vi "Periodic Tasks.vi"() -> ()   [LabVIEW 2011]
doc: "This VI runs in parallel to other tasks. It can contain as many user-defined periodic loops as you need. These can carry out PID or other sorts of timed response."
uses:
  <vilib>/Platform/TimedLoop/XDataNode/timing_clust.ctl
  <vilib>/Platform/TimedLoop/XDataNode/nitl_modes.ctl
  <vilib>/Platform/TimedLoop/XDataNode/wakeup.ctl
  <vilib>/Rock Robotics/WPI/Ultrasonic/WPI_UltrasonicRangeUnits.ctl
  Robot Global Data.vi
  <vilib>/Platform/TimedLoop/XDataNode/XDataNode.xnode
  <vilib>/Platform/TimedLoop/XDataNode/XDNodeRunTimeDep.lvlib
panel:
  out "Angle 2":dbl
  out "Forward Distance":dbl
  in  "pingtime (Sec) 2":sgl=0.5
  out "Angle":dbl
  in  "pingtime (Sec)":sgl=0.5
  out "Ultrasonic Distance":dbl
  # "Outputs"
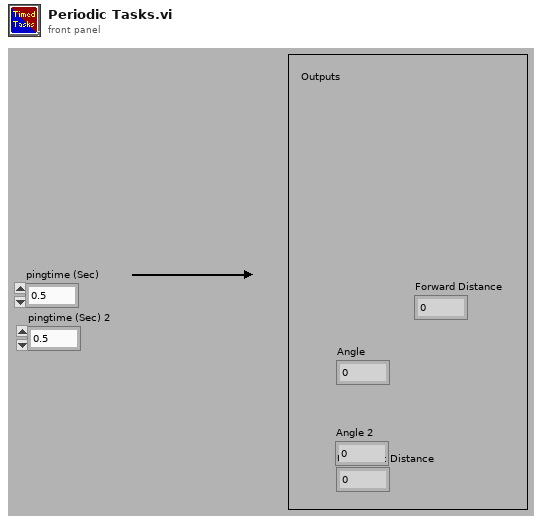
[diagram p1: front panel]
types:
  T1 = typedef "WPI_GyroDevRef.ctl" = cluster{"DevStatus":errorcluster, "Analog Module":T2, "Analog Channel":T3, "Offset":dbl, "Gain (VoltsPerDegree/Second)":dbl}
  T2 = typedef "FPGA_TypedefAnalogModule.ctl" = enum16{"Analog Module 1", "Analog Module 2"}
  T3 = typedef "FPGA_AIChannel.ctl" = enum8{"AI 1", "AI 2", "AI 3", "AI 4", "AI 5", "AI 6", "AI 7", "AI 8", "Invalid"}
  T4 = typedef "WPI_SerialPortRef.ctl" = cluster{"DevStatus":errorcluster, "Serial Port Name":refnum<visa-resource-name>}
  T5 = typedef "WPI_EncoderDevRef.ctl" = cluster{"DevStatus":errorcluster, "EncoderIndex":T6, "CounterIndex":T7, "DistancePerCount":dbl, "Decoding Type":T8}
  T6 = typedef "FPGA_EncoderIdx.ctl" = enum8{"Enc 0", "Enc 1", "Enc 2", "Enc 3", "Invalid"}
  T7 = typedef "FPGA_CounterCtrSystemIndex.ctl" = enum8{"Ctr 0", "Ctr 1", "Ctr 2", "Ctr 3", "Ctr 4", "Ctr 5", "Ctr 6", "Ctr 7", "Invalid"}
  T8 = typedef "WPI_EncoderType.ctl" = enum16{"1x", "2x", "4x"}
  T9 = typedef "WPI_UltrasonicDeviceRef.ctl" = cluster{"DevStatus":errorcluster, "Ping Digital Module":T10, "Echo Digital Module":T10, "Ping Channel":T11, "Echo Channel":T11, "CntIndex":T7}
  T10 = typedef "FPGA_TypedefDigitalModule.ctl" = enum16{"Digital Module 1", "Digital Module 2"}
  T11 = typedef "FPGA_DIOChannel.ctl" = enum8{"DIO 1", "DIO 2", "DIO 3", "DIO 4", "DIO 5", "DIO 6", "DIO 7", "DIO 8", "DIO 9", "DIO 10", "DIO 11", "DIO 12", "DIO 13", "DIO 14", "Invalid"}
  T12 = typedef "WPI_RelayDevRef.ctl" = cluster{"DevStatus":errorcluster, "Relay Channel":T13, "Digital Module":T10, "Relay Direction":T14}
  T13 = typedef "FPGA_DIORelayChannel.ctl" = enum8{"Relay 1", "Relay 2", "Relay 3", "Relay 4", "Relay 5", "Relay 6", "Relay 7", "Relay 8", "Invalid"}
  T14 = typedef "WPI_RelayDirection.ctl" = enum16{"Both directions", "Forward only", "Reverse only"}
  T15 = typedef "XDNodeRunTimeDep.lvlib/timing_clust.ctl" = cluster{"Expected End [f-1]":u64, "Actual End [f-1]":u64, "Finished Late? [f-1]":bool, "Expected End [i-1]":u64, "Actual End [i-1]":u64, "Finished Late? [i-1]":bool, "Expected Start [i]":u64, "Actual Start [i]":u64, "Expected Start [f]":u64, "Actual Start [f]":u64, "Source Name":string, "Structure Name":string, "Period":i64, "Deadline":i64, "Offset":i64, "Start":i64, "Priority":i32, "Timeout":i32, "Mode":T16, "Wakeup Reason":T17, "Error":errorcluster, "Source Type":string, "Secondary Source Type":string, "Global End Time":u64, "Global Start Time":u64, "Frame Duration":u64, "Iteration Duration":u64, "Assigned CPU":i32, "I/O Scan Engine Mode":u32}
  T16 = typedef "XDNodeRunTimeDep.lvlib/nitl_modes.ctl" = enum32{"No Change", "Process missed periods, maintain original phase", "Discard missed periods, maintain original phase", "Process missed periods, ignore original phase", "Discard missed periods, ignore original phase"}
  T17 = typedef "XDNodeRunTimeDep.lvlib/wakeup.ctl" = enum32{"Normal", "Aborted", "Asynchronous wakeup", "Timing source error", "Timed loop error", "Timeout"}
  T18 = typedef "WPI_UltrasonicRangeUnits.ctl" = enum16{"inches", "mm"}
  T19 = cluster{"Driver Station Digital Input (1-8)[0]":bool, "Driver Station Digital Input (1-8)[1]":bool, "Driver Station Digital Input (1-8)[2]":bool, "Driver Station Digital Input (1-8)[3]":bool, "Driver Station Digital Input (1-8)[4]":bool, "Driver Station Digital Input (1-8)[5]":bool, "Driver Station Digital Input (1-8)[6]":bool, "Driver Station Digital Input (1-8)[7]":bool, "Driver Station Digital Input (1-8)[8]":bool}
  T20 = cluster{"Axis 1":dbl, "Axis 2":dbl, "Axis 3":dbl, "Axis 4":dbl, "Axis 5":dbl, "Axis 6":dbl, "Button 1":bool, "Button 2":bool, "Button 3":bool, "Button 4":bool, "Button 5":bool, "Button 6":bool, "Button 7":bool, "Button 8":bool, "Button 9":bool, "Button 10":bool, "Button 11":bool, "Button 12":bool}
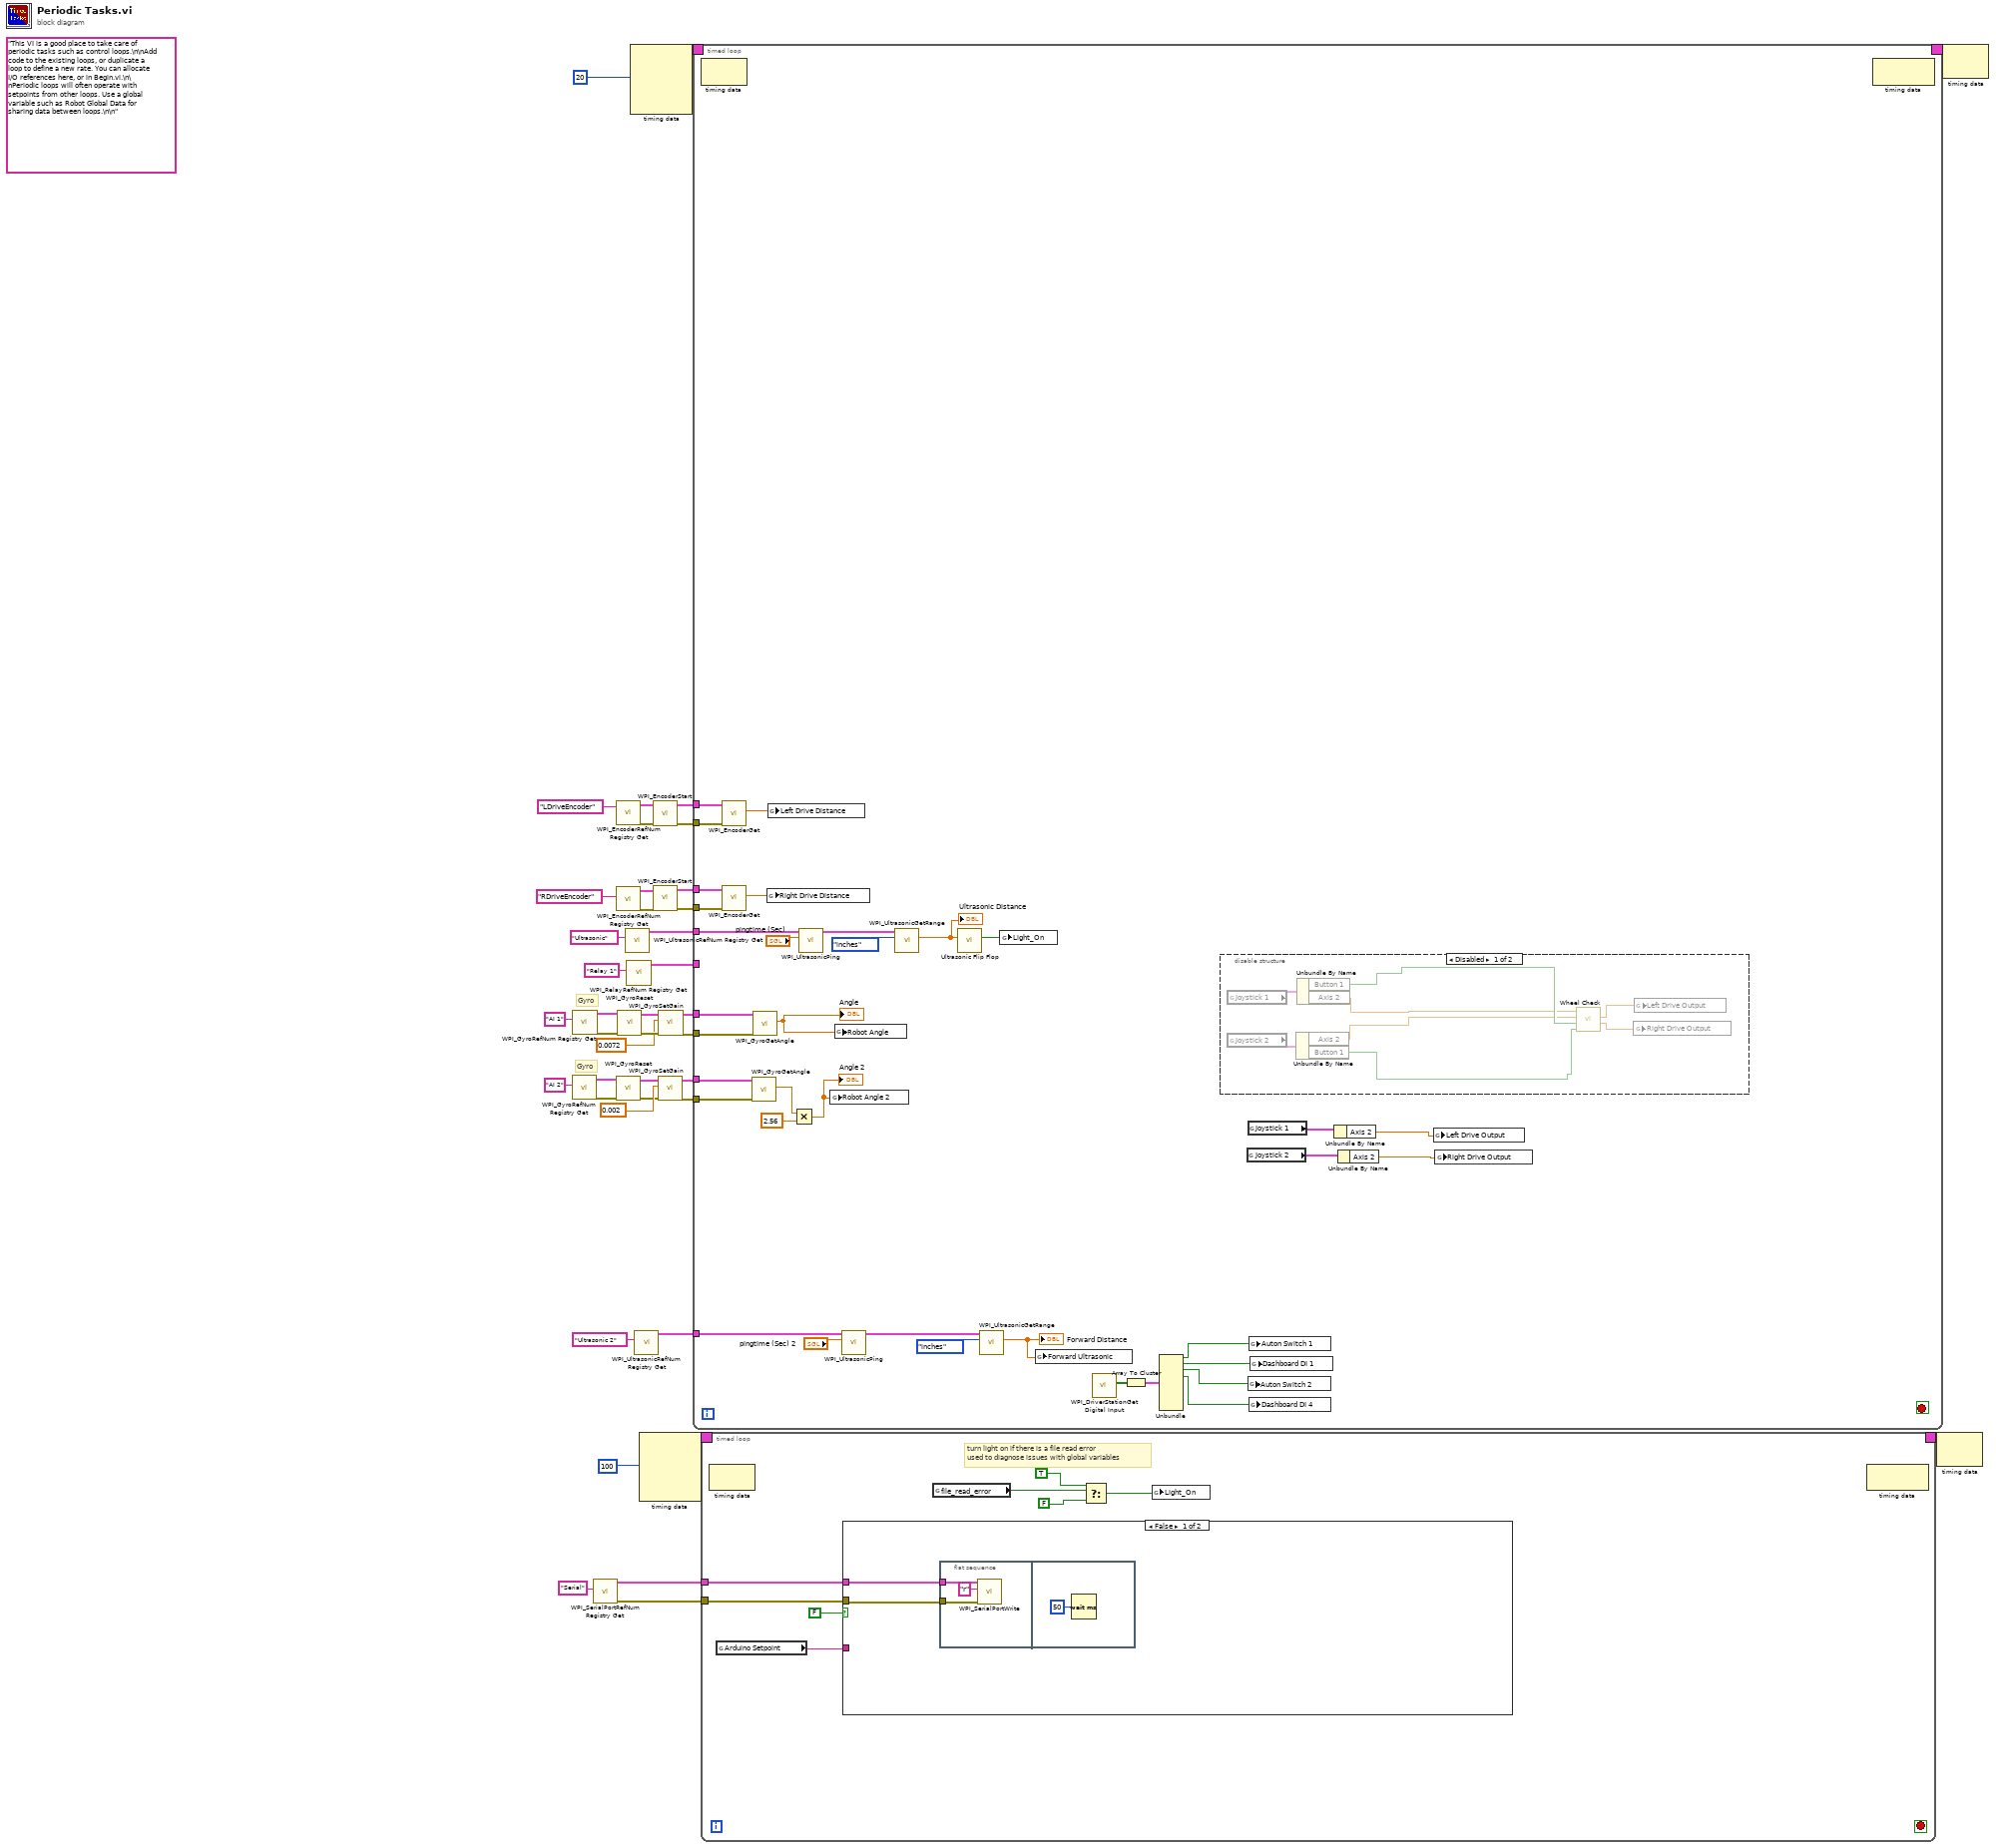
[diagram p0: block diagram]
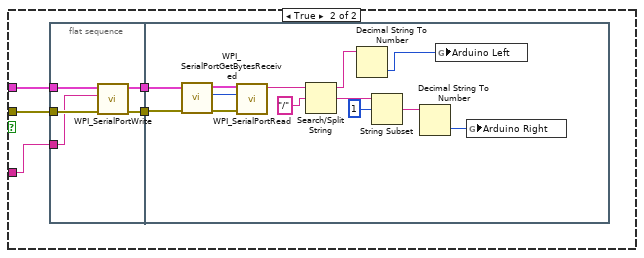
[diagram p2: hidden frame]
diagram:
  (unwired) "This VI is a good place to take care of periodic tasks such as control loops.\n\nAdd code to the existing loops, or duplicate a loop to define a new rate. You can allocate I/O references here, or in Begin.vi.\n\nPeriodic loops will often operate with setpoints from other loops. Use a global variable such as Robot Global Data for sharing data between loops.\n\n"
  # "Gyro"
  # "Gyro"
  n1 = call <vilib>:"WPI_GyroRefNum Registry Get.vi"("refnum name"="AI 2") -> ("error out"=w1:errorcluster, "GyroDevRef"=w8:T1)  [unwired: 1 in, 8 out]
  n2 = call <vilib>:"WPI_GyroRefNum Registry Get.vi"("refnum name"="AI 1") -> ("error out"=w24:errorcluster, "GyroDevRef"=w17:T1)  [unwired: 1 in, 8 out]
  n3 = call <vilib>:"WPI_SerialPortRefNum Registry Get.vi"("refnum name"="Serial") -> ("error out"=w25:errorcluster, "SerialPortRef"=w26:T4)  [unwired: 1 in, 8 out]
  n4 = call <vilib>:"WPI_EncoderRefNum Registry Get.vi"("refnum name"="LDriveEncoder") -> ("error out"=w10:errorcluster, "EncoderDevRef"=w11:T5)  [unwired: 1 in, 8 out]
  n5 = call <vilib>:"WPI_EncoderRefNum Registry Get.vi"("refnum name"="RDriveEncoder") -> ("error out"=w12:errorcluster, "EncoderDevRef"=w13:T5)  [unwired: 1 in, 8 out]
  n6 = call <vilib>:"WPI_GyroReset.vi"("error in (no error)"=w1, "GyroDevRef"=w8) -> ("error out"=w3:errorcluster, "GyroDevRef"=w4:T1)  [unwired: 8 out]
  n7 = call <vilib>:"WPI_GyroReset.vi"("error in (no error)"=w24, "GyroDevRef"=w17) -> ("error out"=w22:errorcluster, "GyroDevRef"=w21:T1)  [unwired: 8 out]
  n8 = call <vilib>:"WPI_UltrasonicRefNum Registry Get.vi"("refnum name"="Ultrasonic") -> ("UltrasonicDevRef"=w28:T9)  [unwired: 1 in, 9 out]
  n9 = call <vilib>:"WPI_RelayRefNum Registry Get.vi"("refnum name"="Relay 1") -> ("RelayDevRef"=w41:T12)  [unwired: 1 in, 9 out]
  n10 = node-c288(i64 20 ("Period")) -> (w39:T15)  [unwired: 3 out]
  n11 = call <vilib>:"WPI_UltrasonicRefNum Registry Get.vi"("refnum name"="Ultrasonic 2") -> ("UltrasonicDevRef"=w16:T9)  [unwired: 1 in, 9 out]
  n12 = node-c288(i64 100 ("Period")) -> (w36:T15)  [unwired: 3 out]
  n13 = call <vilib>:"WPI_EncoderStart.vi"("error in (no error)"=w10, "EncoderDevRef"=w11) -> ("error out"=w33:errorcluster, "EncoderDevRef"=w32:T5)  [unwired: 8 out]
  n14 = call <vilib>:"WPI_EncoderStart.vi"("error in (no error)"=w12, "EncoderDevRef"=w13) -> ("error out"=w30:errorcluster, "EncoderDevRef"=w31:T5)  [unwired: 8 out]
  n15 = call <vilib>:"WPI_GyroSetGain.vi"("error in (no error)"=w3, "Gain (VoltsPerDegree/Second)"=0.002, "GyroDevRef"=w4) -> ("error out"=w6:errorcluster, "GyroDevRef"=w5:T1)  [unwired: 7 out]
  n16 = call <vilib>:"WPI_GyroSetGain.vi"("error in (no error)"=w22, "Gain (VoltsPerDegree/Second)"=0.0072, "GyroDevRef"=w21) -> ("error out"=w19:errorcluster, "GyroDevRef"=w20:T1)  [unwired: 7 out]
  n17 = timed-loop {
    tunnel: w41 -> [_]
    timing: w39 -> [_]
    timing-out: [_] -> w38
    tunnel: w33 -> [w69]
    tunnel: w32 -> [w70]
    tunnel: w30 -> [w67]
    tunnel: w31 -> [w68]
    tunnel: w28 -> [w73]
    tunnel: w20 -> [w66]
    tunnel: w19 -> [w65]
    tunnel: w16 -> [w60]
    tunnel: w5 -> [w49]
    tunnel: w6 -> [w50]
    stop <- _ stop-if-true
    n18 = node-c288() -> ()  [unwired: 2 out]
    n19 = call <vilib>:"WPI_EncoderGet.vi"("error in (no error)"=w69, "EncoderDevRef"=w70) -> ("Distance"=w76:dbl)  [unwired: 9 out]
    n20 = call <vilib>:"WPI_EncoderGet.vi"("error in (no error)"=w67, "EncoderDevRef"=w68) -> ("Distance"=w75:dbl)  [unwired: 9 out]
    n21 = call <vilib>:"WPI_GyroGetAngle.vi"("error in (no error)"=w50, "GyroDevRef"=w49) -> ("Angle"=w47:dbl)  [unwired: 9 out]
    n22 = call <vilib>:"WPI_GyroGetAngle.vi"("error in (no error)"=w65, "GyroDevRef"=w66) -> ("Angle"=w64:dbl)  [unwired: 9 out]
    "Angle" <- w64
    n23 = global write "Robot Global Data.vi" "Right Drive Distance"(w75) -> ()
    n24 = global write "Robot Global Data.vi" "Left Drive Distance"(w76) -> ()
    n25 = Multiply(x=w47, y=2.56) -> (x*y=w46:dbl)
    "Angle 2" <- w46
    n26 = call <vilib>:"WPI_UltrasonicPing.vi"("pingtime (Sec)"="pingtime (Sec)", "UltrasonicDevRef"=w73) -> ("UltrasonicDevRef"=w72:T9)  [unwired: 1 in, 8 out]
    n27 = global write "Robot Global Data.vi" "Robot Angle 2"(w46) -> ()
    n28 = global write "Robot Global Data.vi" "Robot Angle"(w64) -> ()
    n29 = call <vilib>:"WPI_UltrasonicPing.vi"("pingtime (Sec)"="pingtime (Sec) 2", "UltrasonicDevRef"=w60) -> ("UltrasonicDevRef"=w61:T9)  [unwired: 1 in, 8 out]
    n30 = call <vilib>:"WPI_UltrasonicGetRange.vi"("Range Units"=WPI_UltrasonicRangeUnits."inches", "UltrasonicDevRef"=w72) -> ("Distance"=w63:dbl)  [unwired: 1 in, 8 out]
    "Ultrasonic Distance" <- w63
    n31 = call "Ultrasonic Flip Flop.vi"("Distance"=w63) -> ("output"=w57:bool)  [unwired: 10 out]
    n32 = call <vilib>:"WPI_UltrasonicGetRange.vi"("Range Units"=WPI_UltrasonicRangeUnits."inches", "UltrasonicDevRef"=w61) -> ("Distance"=w58:dbl)  [unwired: 1 in, 8 out]
    "Forward Distance" <- w58
    n33 = global write "Robot Global Data.vi" "Light_On"(w57) -> ()
    n34 = global write "Robot Global Data.vi" "Forward Ultrasonic"(w58) -> ()
    n35 = call <vilib>:"WPI_DriverStationGet Digital Input.vi"() -> ("Driver Station Digital Input (1-8)"=w53:bool[])  [unwired: 11 out]
    n36 = Array To Cluster(array=w53) -> (cluster=w54:T19)
    n37 = Unbundle(w54) -> ("Driver Station Digital Input (1-8)[0]"=w55:bool, "Driver Station Digital Input (1-8)[1]"=w51:bool, "Driver Station Digital Input (1-8)[2]"=w56:bool, "Driver Station Digital Input (1-8)[3]"=w52:bool)  [unwired: 5 out]
    n38 = disable-structure shown="Disabled" {
      frame Disabled {
        n39 = global read "Robot Global Data.vi" "Joystick 1"() -> (w83:T20)
        n40 = global read "Robot Global Data.vi" "Joystick 2"() -> (w84:T20)
        n41 = Unbundle By Name(w84) -> ("Axis 2"=w77:dbl, "Button 1"=w80:bool)
        n42 = Unbundle By Name(w83) -> ("Button 1"=w79:bool, "Axis 2"=w78:dbl)
        n43 = call "Wheel Check.vi"("Trigger 2"=w80, "Trigger 1"=w79, "Right Drive"=w77, "Left Drive"=w78) -> ("Right Out"=w81:dbl, "Left Out"=w82:dbl)  [unwired: 6 out]
        n44 = global write "Robot Global Data.vi" "Right Drive Output"(w81) -> ()
        n45 = global write "Robot Global Data.vi" "Left Drive Output"(w82) -> ()
      }
      frame Enabled {
      }
    }
    n46 = global read "Robot Global Data.vi" "Joystick 2"() -> (w44:T20)
    n47 = global read "Robot Global Data.vi" "Joystick 1"() -> (w45:T20)
    n48 = global write "Robot Global Data.vi" "Auton Switch 2"(w56) -> ()
    n49 = global write "Robot Global Data.vi" "Auton Switch 1"(w55) -> ()
    n50 = global write "Robot Global Data.vi" "Dashboard DI 4"(w52) -> ()
    n51 = global write "Robot Global Data.vi" "Dashboard DI 1"(w51) -> ()
    n52 = Unbundle By Name(w45) -> ("Axis 2"=w42:dbl)
    n53 = Unbundle By Name(w44) -> ("Axis 2"=w43:dbl)
    n54 = global write "Robot Global Data.vi" "Left Drive Output"(w42) -> ()
    n55 = global write "Robot Global Data.vi" "Right Drive Output"(w43) -> ()
    n56 = node-c288() -> ()  [unwired: 2 out]
  }
  n57 = timed-loop {
    timing: w36 -> [_]
    timing-out: [_] -> w35
    tunnel: w26 -> [w93]
    tunnel: w25 -> [w92]
    stop <- _ stop-if-true
    # "turn light on if there is a file read error\nused to diagnose issues with global variables"
    n58 = node-c288() -> ()  [unwired: 2 out]
    n59 = global read "Robot Global Data.vi" "Arduino Setpoint"() -> (w94:string)
    n60 = case shown="False" FALSE {
      tunnel: w93 -> [w96 w105]
      tunnel: w92 -> [w95 w104]
      tunnel: w94 -> [_ w103]
      frame False {
        n61 = flat-sequence {
          tunnel: w96 -> [w99]
          tunnel: w95 -> [w98]
          frame #0 {
            n62 = call <vilib>:"WPI_SerialPortWrite.vi"("error in (no error)"=w98, "Buffer"="r", "SerialPortRef"=w99) -> ()  [unwired: 9 out]
          }
          frame #1 {
            n63 = Wait (ms)(milliseconds to wait=u32 50) -> ()  [unwired: 1 out]
          }
        }
      }
      frame True {
        n64 = flat-sequence {
          tunnel: w105 -> [w110]
          tunnel: w104 -> [w109]
          tunnel: [w108] -> w102
          tunnel: [w107] -> w101
          tunnel: w103 -> [w106]
          tunnel: w102 -> [w115]
          tunnel: w101 -> [w114]
          frame #0 {
            n65 = call <vilib>:"WPI_SerialPortWrite.vi"("error in (no error)"=w109, "Buffer"=w106, "SerialPortRef"=w110) -> ("error out"=w107:errorcluster, "SerialPortRef"=w108:T4)  [unwired: 7 out]
          }
          frame #1 {
            n66 = call <vilib>:"WPI_SerialPortGetBytesReceived.vi"("error in (no error)"=w114, "SerialPortRef"=w115) -> ("error out"=w111:errorcluster, "Bytes at Port"=w112:u32, "SerialPortRef"=w113:T4)  [unwired: 7 out]
            n67 = call <vilib>:"WPI_SerialPortRead.vi"("error in (no error)"=w111, "Num Bytes to Read"=w112, "SerialPortRef"=w113) -> ("Buffer"=w118:string)  [unwired: 8 out]
            n68 = Search/Split String(string=w118, search string/char (-)="/") -> (substring before match=w120:string, match + rest of string=w122:string)  [unwired: 2 out]
            n69 = Decimal String To Number(string=w120) -> (number=w117:i32)  [unwired: 3 out]
            n70 = String Subset(string=w122, offset (0)=1) -> (substring=w119:string)  [unwired: 1 out]
            n71 = Decimal String To Number(string=w119) -> (number=w116:i32)  [unwired: 3 out]
            n72 = global write "Robot Global Data.vi" "Arduino Left"(w117) -> ()
            n73 = global write "Robot Global Data.vi" "Arduino Right"(w116) -> ()
          }
        }
      }
    }
    n74 = global read "Robot Global Data.vi" "file_read_error"() -> (w90:bool)
    n75 = Select(t=TRUE, s=w90, f=FALSE) -> (s? t:f=w89:bool)
    n76 = global write "Robot Global Data.vi" "Light_On"(w89) -> ()
    n77 = node-c288() -> ()  [unwired: 2 out]
  }
  n78 = node-c288(w35) -> ()  [unwired: 1 out]
  n79 = node-c288(w38) -> ()  [unwired: 1 out]
